vi "UART_ExternalSupply.vi"(7 "Settling (s)":dbl=0.2 format="%#_13g", 8 "error in (no error)":errorcluster, 9 "voltage level (V)":dbl=5.0 format="%#_13g", 10 "Supply Pin":string="Vext5", 11 "IVI Refnum in":refnum<k15>) -> (0 "error out":errorcluster, 3 "IVI Refnum out":refnum<k15>)   [LabVIEW 2024, in "UART.lvlib"]
doc: "Set one pin to PPMU mode suppling voltage to the DUT.\nAfter staring sourcing, a setling time is applied to make sure the DUT firmware starts properly"
uses:
  <instrlib>/niDigital/niDigital.llb/niDigital Selected Function.ctl
  <instrlib>/niDigital/niDigital.llb/niDigital Output Function.ctl
  UART.lvlib
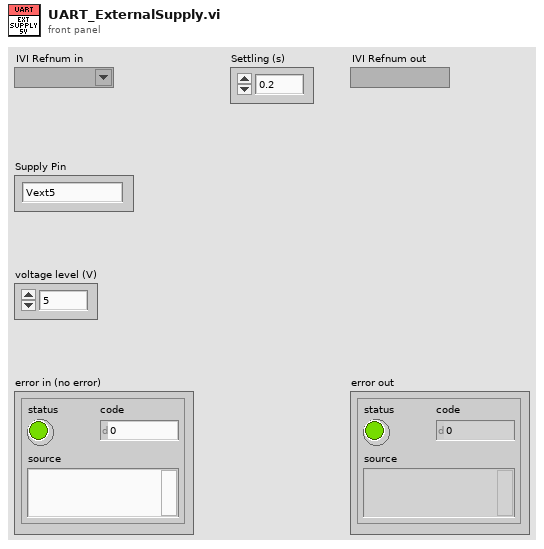
[diagram p1: front panel]
types:
  T1 = typedef "niDigital Output Function.ctl" = i32
  T2 = typedef "niDigital Selected Function.ctl" = i32
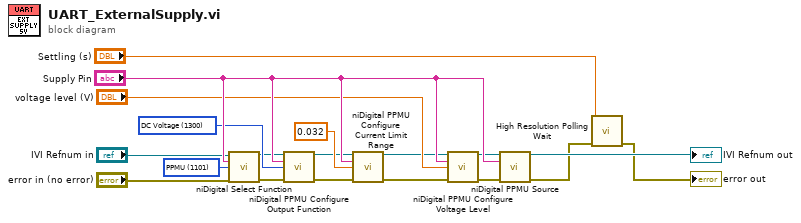
[diagram p0: block diagram]
diagram:
  w6 = T1 1300 items=["DC Voltage"=1300, "DC Current"=1301] ("output function")
  w3 = T2 1101 items=["Digital"=1100, "PPMU"=1101, "Off"=1102, "Disconnect"=1103, "RIO"=1104] ("function")
  n1 = call <instrlib>:"niDigital Select Function.vi"("instrument handle"="IVI Refnum in", "channel list"="Supply Pin", "function"=w3, "error in"="error in (no error)") -> ("instrument handle out"=w4:refnum<k15>, "error out"=w5:errorcluster)  [unwired: 10 in]
  n2 = call <instrlib>:"niDigital PPMU Configure Output Function.vi"("instrument handle"=w4, "channel list"="Supply Pin", "output function"=w6, "error in"=w5) -> ("instrument handle out"=w8:refnum<k15>, "error out"=w7:errorcluster)  [unwired: 10 in]
  n3 = call <instrlib>:"niDigital PPMU Configure Current Limit Range.vi"("instrument handle"=w8, "channel list"="Supply Pin", "current limit range (A)"=0.032, "error in"=w7) -> ("instrument handle out"=w10:refnum<k15>, "error out"=w9:errorcluster)  [unwired: 10 in]
  n4 = call <instrlib>:"niDigital PPMU Configure Voltage Level.vi"("instrument handle"=w10, "channel list"="Supply Pin", "voltage level (V)"="voltage level (V)", "error in"=w9) -> ("instrument handle out"=w13:refnum<k15>, "error out"=w14:errorcluster)  [unwired: 10 in]
  n5 = call <instrlib>:"niDigital PPMU Source.vi"("instrument handle"=w13, "channel list"="Supply Pin", "error in"=w14) -> ("instrument handle out"=→"IVI Refnum out":refnum<k15>, "error out"=w17:errorcluster)  [unwired: 11 in]
  n6 = call <vilib>:"High Resolution Polling Wait.vi"("error in (no error)"=w17, "seconds to wait"="Settling (s)") -> ("error out"=→"error out":errorcluster)  [unwired: 9 in]
